vi "recipe_logic.vi"(5 "change_in_event":refnum<user-event>, 7 "transition_queue":refnum<queue>, 8 "error in (no error)":errorcluster, 11 "data_in":T1) -> (0 "error out":errorcluster, 1 "data out":variant, 2 "change":bool, 3 "data_out":T1)   [LabVIEW 2015, in "lv-recipe-machine.lvlib"]
uses:
  lv-recipe-machine.lvlib
  public/_controls/recipe_data.ctl
  public/_controls/mode.ctl
  public/_controls/manual_state.ctl
  public/_controls/automatic_state.ctl
  public/_controls/timer.ctl
  public/_controls/recipe_step.ctl
  public/_controls/change.ctl
  public/_controls/transition.ctl
  _controls/timers.ctl
  _controls/timer_command.ctl
  public/_controls/step.ctl
  public/_controls/error.ctl
  _controls/automatic_vi_variant_data.ctl
  <vilib>/ptbypt/NI_PtbyPt.lvlib
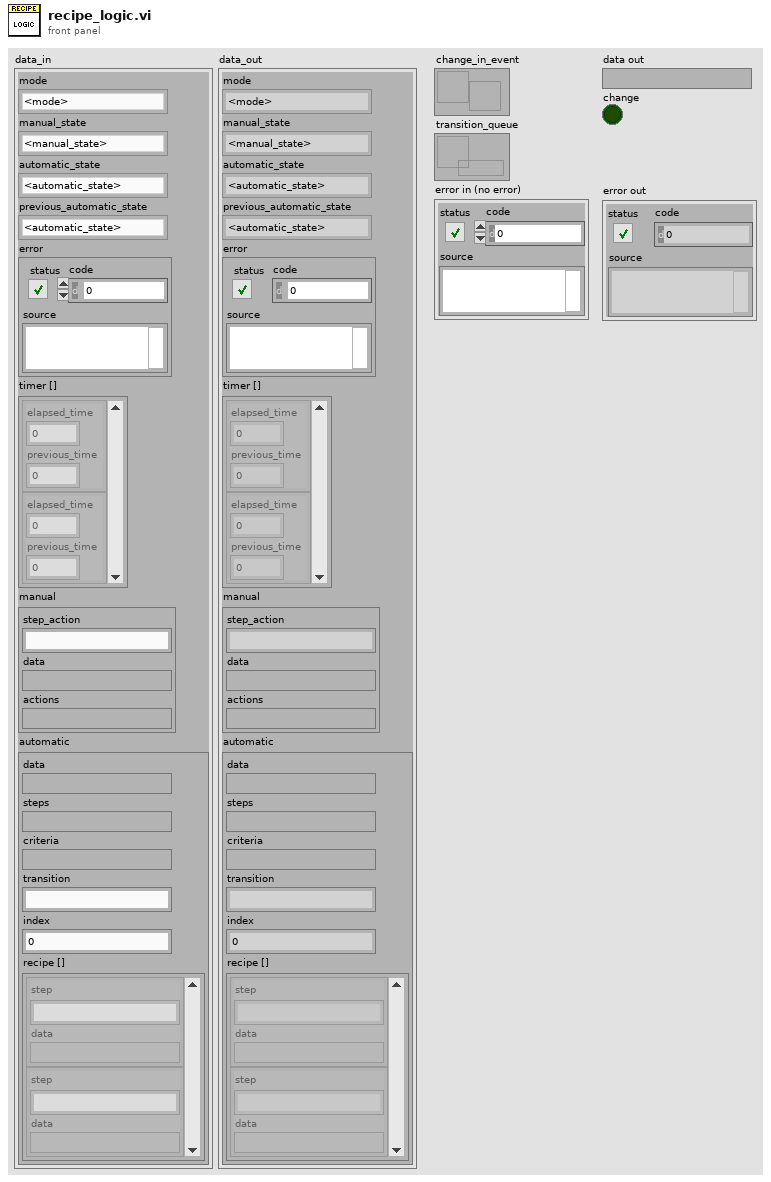
[diagram p1: front panel]
types:
  T1 = typedef "lv-recipe-machine.lvlib/recipe_data.ctl" = cluster{"mode":T2, "manual_state":T3, "automatic_state":T4, "previous_automatic_state":T4, "error":errorcluster, "timer []":T5[], "manual":cluster{"step_action":string, "data":variant, "actions":variant}, "automatic":cluster{"data":variant, "steps":variant, "criteria":variant, "transition":string, "index":i32, "recipe []":T6[]}}
  T2 = typedef "lv-recipe-machine.lvlib/mode.ctl" = enum16{"<mode>", "manual", "automatic", "<null>"}
  T3 = typedef "lv-recipe-machine.lvlib/manual_state.ctl" = enum16{"<manual_state>", "failed", "action", "running", "idle", "<null>"}
  T4 = typedef "lv-recipe-machine.lvlib/automatic_state.ctl" = enum16{"<automatic_state>", "failed", "idle", "running", "paused", "stopped", "<null>"}
  T5 = typedef "lv-recipe-machine.lvlib/timer.ctl" = cluster{"elapsed_time":dbl, "previous_time":dbl}
  T6 = typedef "lv-recipe-machine.lvlib/recipe_step.ctl" = cluster{"step":string, "data":variant}
  T7 = typedef "lv-recipe-machine.lvlib/timers.ctl" = enum16{"<timers>", "step", "recipe", "<null>"}
  T8 = typedef "lv-recipe-machine.lvlib/timer_command.ctl" = enum16{"<timer_command>", "start", "read", "pause", "resume", "stop", "<null>"}
  T9 = typedef "lv-recipe-machine.lvlib/automatic_vi_variant_data.ctl" = cluster{"current_state":T4, "previous_state":T4, "criteria":variant, "data":variant, "recipe_data":variant, "index":i32, "step":string, "steps":variant}
  T10 = typedef "lv-recipe-machine.lvlib/error.ctl" = enum16{"<error>", "bad_command", "command_queue_timeout", "stop_notifier_timeout", "die_command_timeout", "not_in_manual_mode", "not_in_automatic_mode", "not_in_automatic_idle", "not_in_automatic_running", "not_in_automatic_paused", "automatic_step_not_found", "manual_action_not_found", "automatic_not_transition_vi", "transition_step_not_found", "unsupported_vi_type", "<null>"}
  T11 = typedef "lv-recipe-machine.lvlib/step.ctl" = cluster{"name":string, "data":variant, "vi_reference":variant}
  T12 = cluster{"data":variant, "steps":variant, "criteria":variant, "transition":string, "index":i32, "recipe []":T6[]}
  T13 = cluster{"step_action":string, "data":variant, "actions":variant}
  T14 = typedef "lv-recipe-machine.lvlib/transition.ctl" = cluster{"next_index":i32, "data":variant, "recipe_data":variant, "error":errorcluster}
  T15 = cluster{"recipe_data out":variant, "error":errorcluster}
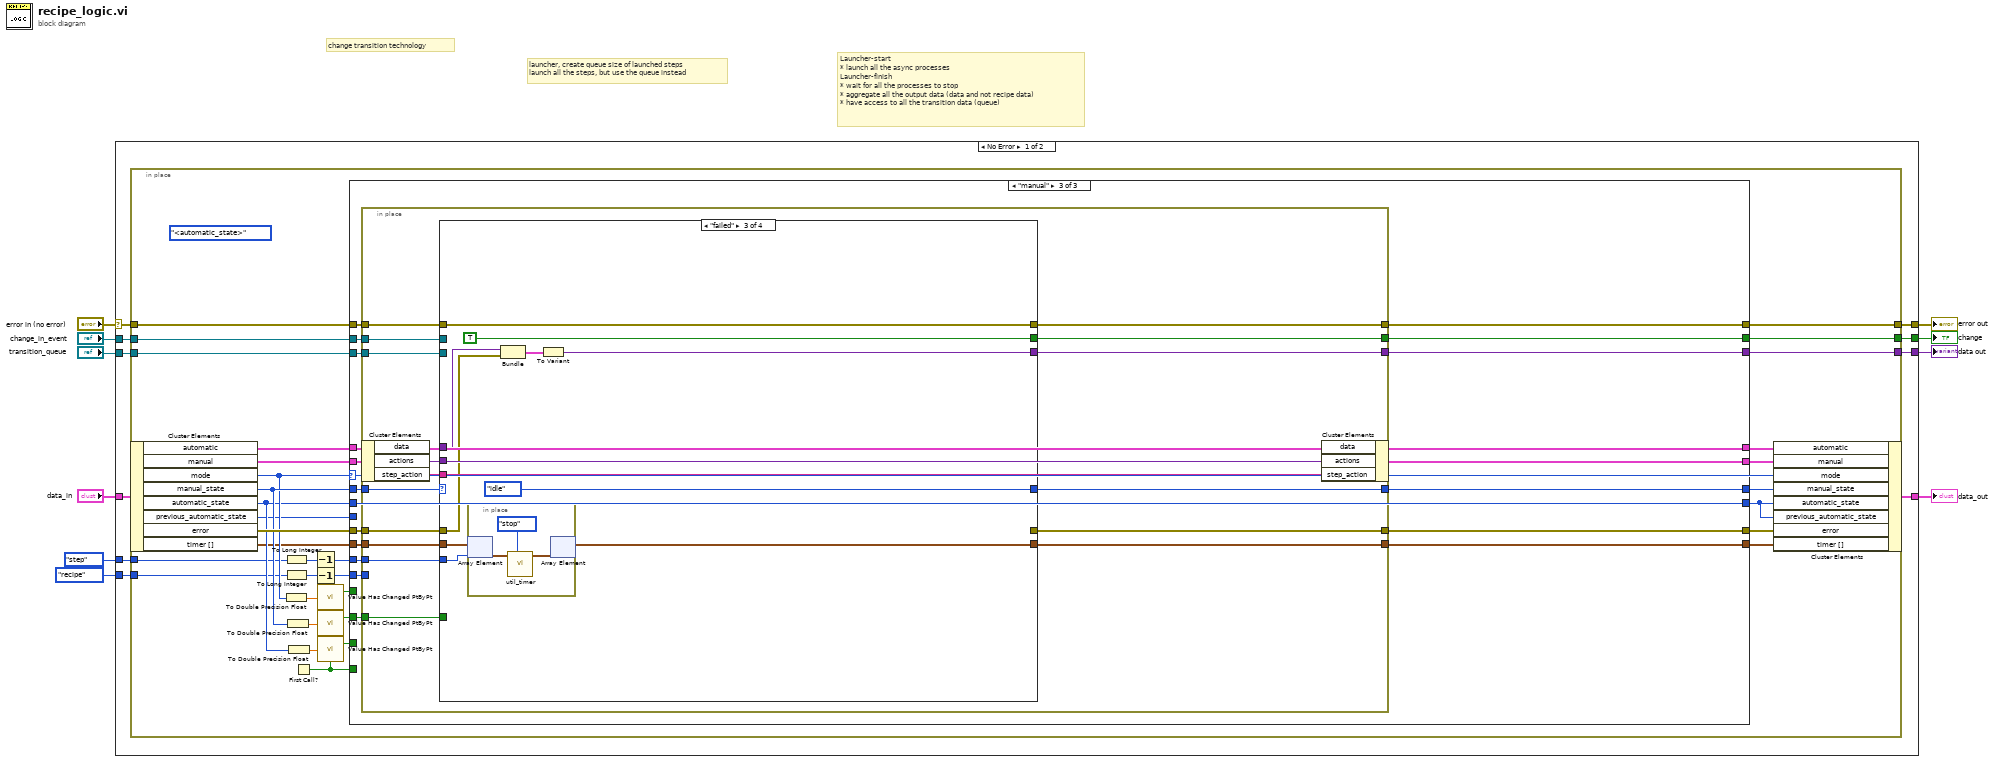
[diagram p0: block diagram]
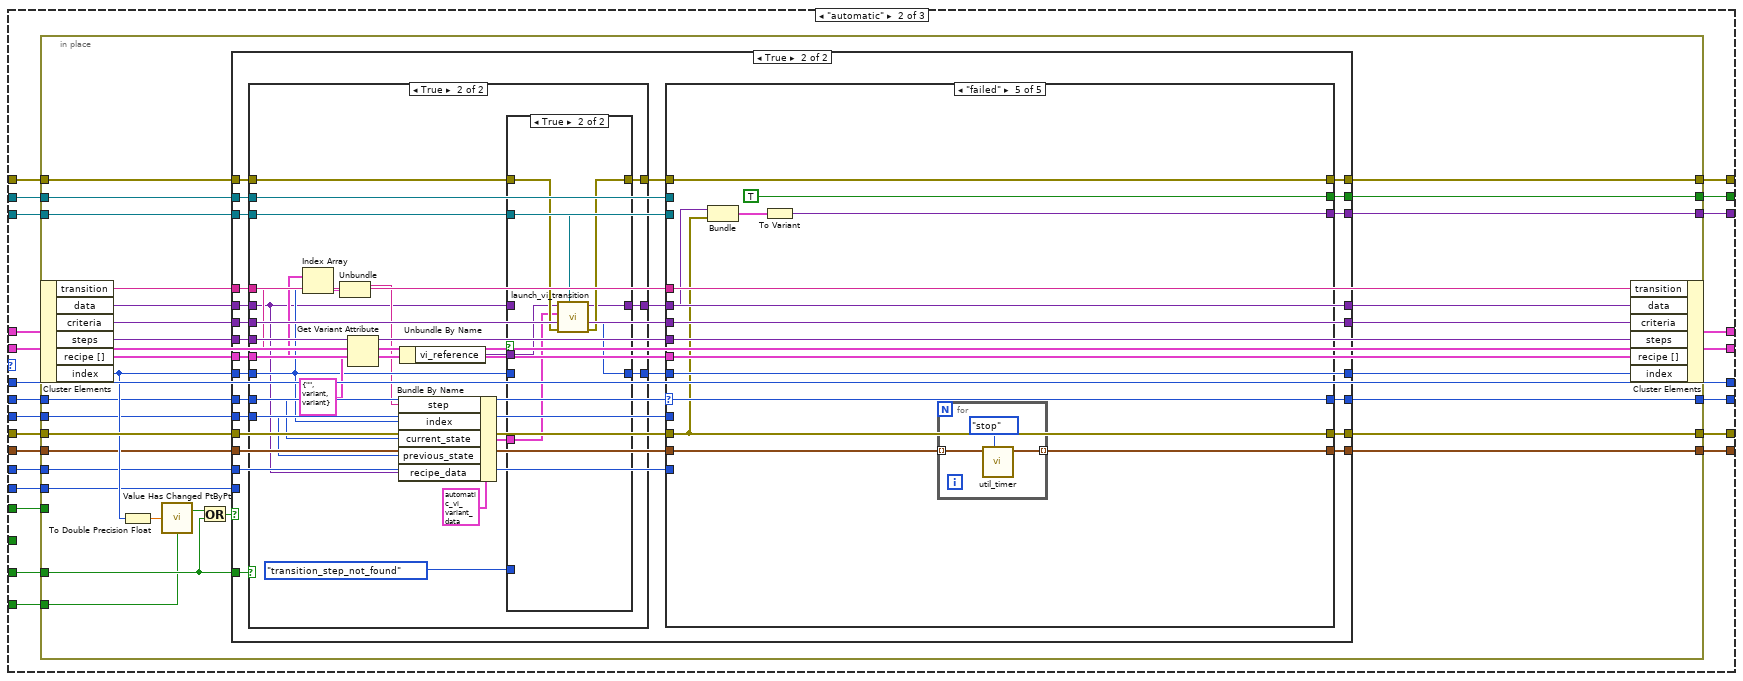
[diagram p3: hidden frame]
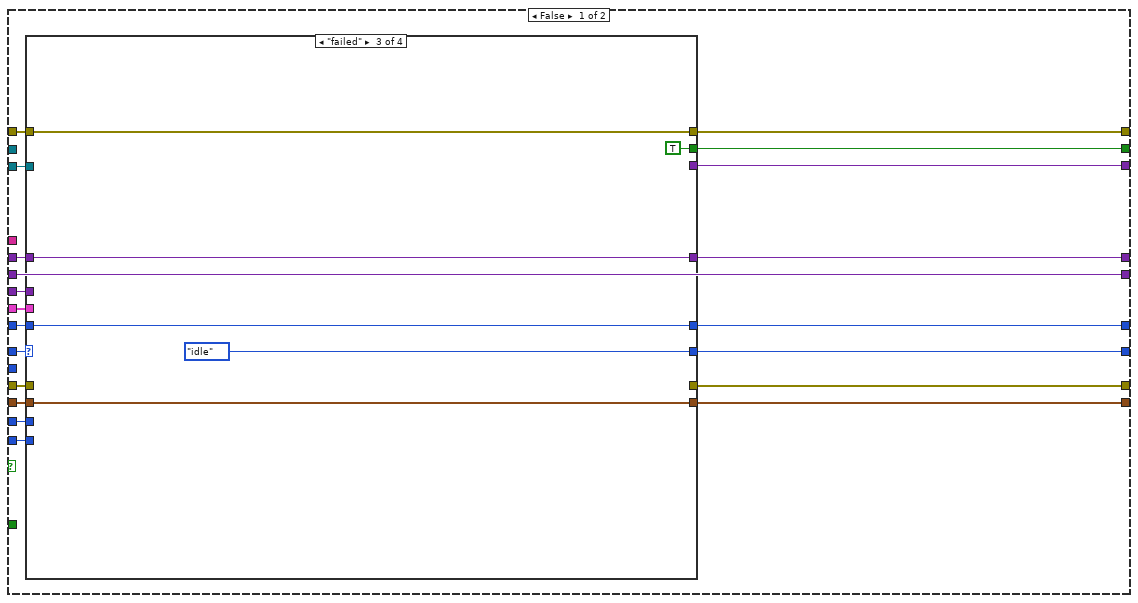
[diagram p4: hidden frame]
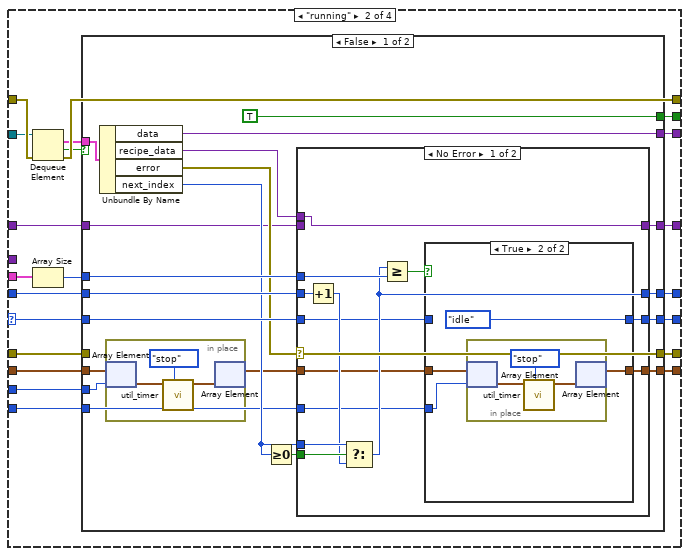
[diagram p6: hidden frame]
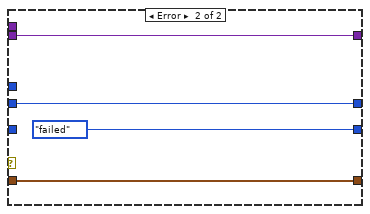
[diagram p8: hidden frame]
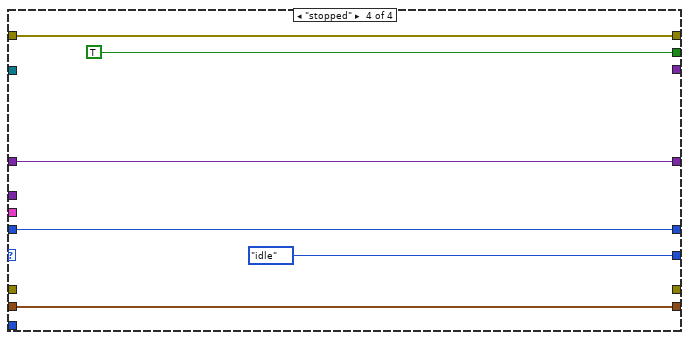
[diagram p10: hidden frame]
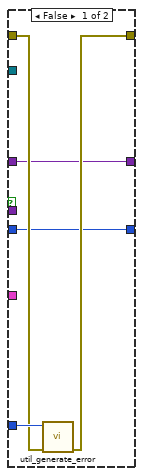
[diagram p12: hidden frame]
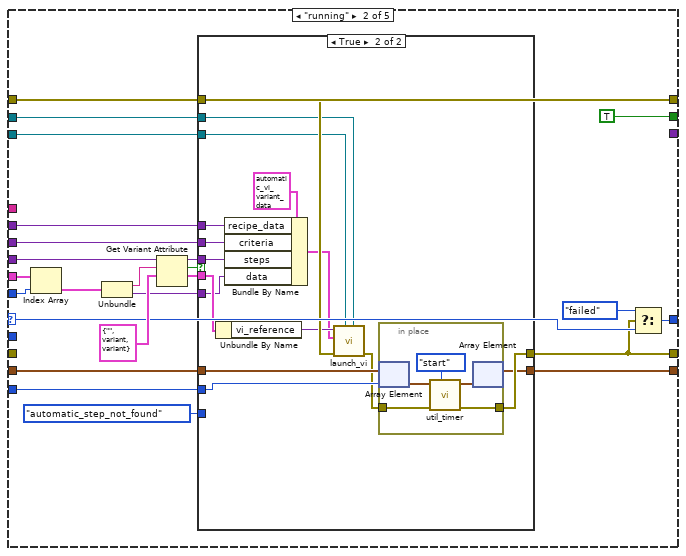
[diagram p14: hidden frame]
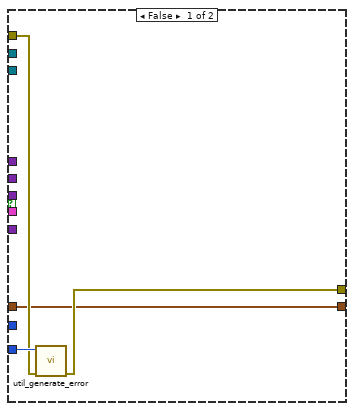
[diagram p15: hidden frame]
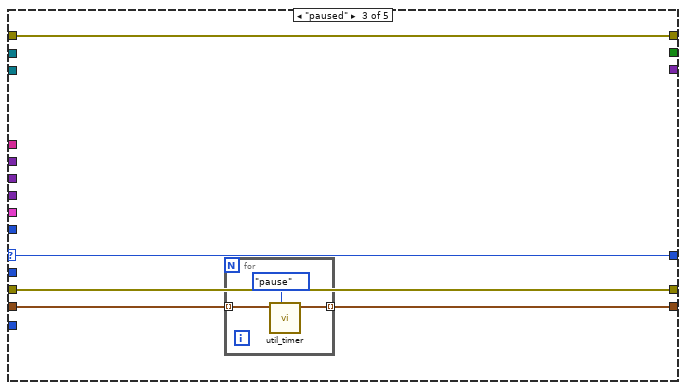
[diagram p16: hidden frame]
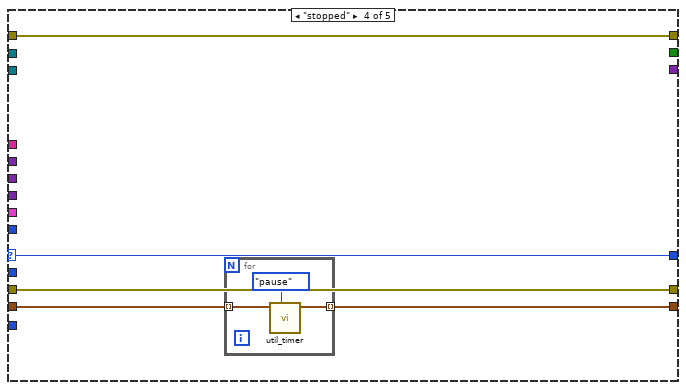
[diagram p17: hidden frame]
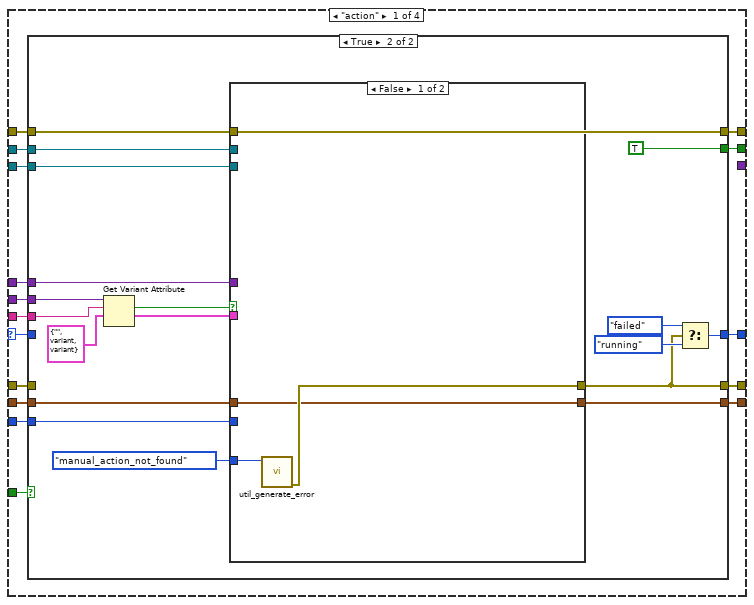
[diagram p18: hidden frame]
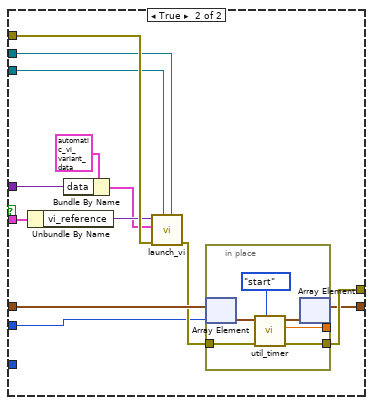
[diagram p20: hidden frame]
diagram:
  # "change transition technology"
  # "launcher, create queue size of launched steps\nlaunch all the steps, but use the queue instead"
  # "Launcher-start\n* launch all the async processes\nLauncher-finish\n* wait for all the processes to stop\n* aggregate all the output data (data and not recipe data)\n* have access to all the transition data (queue)"
  n1 = case shown="No Error" "error in (no error)" {
    selector: "error in (no error)" -> [w20 w512]
    tunnel: [w17 w512] -> w9
    tunnel: "data_in" -> [w19 w511]
    tunnel: [w18 w511] -> w7
    tunnel: [w16 _] -> w6
    tunnel: [w15 _] -> w5
    tunnel: "change_in_event" -> [w14 _]
    tunnel: "transition_queue" -> [w13 _]
    tunnel: timers."step" ("timers") -> [w12 _]
    tunnel: timers."recipe" ("timers") -> [w11 _]
    frame No Error {
      n2 = in-place {
        in-place-border: w20 -> [w46]
        in-place-border: [w43] -> w17
        in-place-border: [w40] -> w16
        in-place-border: [w39] -> w15
        in-place-border: w14 -> [w30]
        in-place-border: w13 -> [w29]
        in-place-border: w12 -> [w24]
        in-place-border: w11 -> [w23]
        (unwired) automatic_state."<automatic_state>" ("automatic_state")
        n3 = in-place-cluster #1(w19) -> ("automatic"=w35:T12, "manual"=w34:T13, "mode"=w42:T2, "manual_state"=w44:T3, "automatic_state"=w38:T4, "previous_automatic_state"=w37:T4, "error"=w53:errorcluster, "timer []"=w28:T5[])
        n4 = To Long Integer(number=w24) -> (32bit integer=w21:i32)
        n5 = To Long Integer(number=w23) -> (32bit integer=w22:i32)
        n6 = To Double Precision Float(number=w42) -> (double precision float=w52:dbl)
        n7 = To Double Precision Float(number=w44) -> (double precision float=w51:dbl)
        n8 = To Double Precision Float(number=w38) -> (double precision float=w50:dbl)
        n9 = First Call?() -> (First Call?: T/F=w45:bool)
        n10 = Decrement(x=w21) -> (x-1=w26:i32)
        n11 = Decrement(x=w22) -> (x-1=w25:i32)
        n12 = call <vilib>:"Value Has Changed PtByPt.vi"("input data point"=w52, "initialize"=w45) -> ("has changed"=w49:bool)  [unwired: 1 out]
        n13 = call <vilib>:"Value Has Changed PtByPt.vi"("input data point"=w51, "initialize"=w45) -> ("has changed"=w48:bool)  [unwired: 1 out]
        n14 = call <vilib>:"Value Has Changed PtByPt.vi"("input data point"=w50, "initialize"=w45) -> ("has changed"=w47:bool)  [unwired: 1 out]
        n15 = case shown="\"manual\"" w42 {
          tunnel: w44 -> [w59 w78 w383]
          tunnel: w38 -> [w58 w81 w378]
          tunnel: w49 -> [_ w61 _]
          tunnel: w48 -> [_ _ w382]
          tunnel: w47 -> [_ w77 _]
          tunnel: w45 -> [_ w74 _]
          tunnel: w46 -> [w60 w80 w381]
          tunnel: [w60 w79 w380] -> w43
          tunnel: [w59 w78 w379] -> w41
          tunnel: [w58 w71 w378] -> w31
          tunnel: [_ w73 w377] -> w40
          tunnel: [_ w72 w376] -> w39
          tunnel: w34 -> [w57 w82 w374]
          tunnel: w35 -> [w56 w76 w375]
          tunnel: [w56 w75 w375] -> w32
          tunnel: [w57 w82 w373] -> w33
          tunnel: w37 -> [_ w68 _]
          tunnel: w53 -> [w55 w70 w372]
          tunnel: [w55 w69 w371] -> w36
          tunnel: w30 -> [_ w67 w369]
          tunnel: w29 -> [_ w66 w370]
          tunnel: w28 -> [w54 w65 w366]
          tunnel: [w54 w62 w365] -> w27
          tunnel: w26 -> [_ w64 w368]
          tunnel: w25 -> [_ w63 w367]
          frame Default {
          }
          frame "automatic" {
            n16 = in-place {
              in-place-border: w81 -> [w90]
              in-place-border: w80 -> [w111]
              in-place-border: [w110] -> w79
              in-place-border: w77 -> [w92]
              in-place-border: w74 -> [w84]
              in-place-border: [w104] -> w73
              in-place-border: [w103] -> w72
              in-place-border: [w102] -> w71
              in-place-border: w70 -> [w99]
              in-place-border: [w98] -> w69
              in-place-border: w68 -> [w93]
              in-place-border: w67 -> [w89]
              in-place-border: w66 -> [w88]
              in-place-border: w65 -> [w87]
              in-place-border: w64 -> [w86]
              in-place-border: w63 -> [w85]
              in-place-border: [w83] -> w62
              in-place-border: w61 -> [_]
              n17 = in-place-cluster #2(w76) -> ("transition"=w94:string, "data"=w101:variant, "criteria"=w97:variant, "steps"=w107:variant, "recipe []"=w109:T6[], "index"=w96:i32)
              n18 = To Double Precision Float(number=w96) -> (double precision float=w108:dbl)
              n19 = call <vilib>:"Value Has Changed PtByPt.vi"("input data point"=w108, "initialize"=w84) -> ("has changed"=w106:bool)  [unwired: 1 out]
              n20 = Or(x=w106, y=w92) -> (x .or. y?=w105:bool)
              n21 = case shown="True" w105 {
                tunnel: w90 -> [w131 w238]
                tunnel: w111 -> [w130 w243]
                tunnel: [w129 w247] -> w110
                tunnel: w107 -> [w119 w236]
                tunnel: w96 -> [w128 w234]
                tunnel: w109 -> [w127 w230]
                tunnel: [w126 w246] -> w104
                tunnel: [w125 w224] -> w103
                tunnel: [w124 w245] -> w102
                tunnel: w101 -> [w123 w240]
                tunnel: [w122 w235] -> w100
                tunnel: w99 -> [w121 w233]
                tunnel: [w120 w244] -> w98
                tunnel: w97 -> [w118 w239]
                tunnel: [w118 w239] -> w95
                tunnel: w94 -> [_ w242]
                tunnel: w93 -> [_ w237]
                tunnel: w92 -> [_ w232]
                tunnel: [w117 w231] -> w91
                tunnel: w89 -> [_ w229]
                tunnel: w88 -> [w116 w228]
                tunnel: w87 -> [w115 w227]
                tunnel: w86 -> [w113 w226]
                tunnel: w85 -> [w112 _]
                tunnel: [w114 w225] -> w83
                frame False {
                  n22 = case shown="\"failed\"" w131 {
                    selector: w131 -> [w136 w153 _ _]
                    tunnel: w130 -> [w137 w158 w214 w223]
                    tunnel: [w137 w157 w214 w223] -> w129
                    tunnel: w119 -> [_ _ _ _]
                    tunnel: w128 -> [w133 w151 w215 w219]
                    tunnel: w127 -> [_ w150 _ _]
                    tunnel: [_ w155 TRUE TRUE] -> w126
                    tunnel: [_ w154 _ _] -> w125
                    tunnel: [w136 w152 automatic_state."idle" ("automatic_state") automatic_state."idle" ("automatic_state")] -> w124
                    tunnel: w123 -> [w135 w148 w216 w220]
                    tunnel: [w135 w147 w216 w220] -> w122
                    tunnel: w121 -> [w134 w156 _ _]
                    tunnel: [w134 w146 _ _] -> w120
                    tunnel: [w133 w145 w215 w219] -> w117
                    tunnel: w116 -> [_ w142 _ _]
                    tunnel: w115 -> [w132 w141 w213 w218]
                    tunnel: [w132 w139 w213 w218] -> w114
                    tunnel: w113 -> [_ w140 _ _]
                    tunnel: w112 -> [_ w138 _ _]
                    frame Default {
                    }
                    frame "running" {
                      n23 = Dequeue Element(queue=w142, error in (no error)=w158) -> (element=w144:T14, timed out?=w143:bool, error out=w157:errorcluster)  [unwired: 1 in, 1 out]
                      n24 = Array Size(array=w150) -> (size(s)=w149:i32)
                      n25 = case shown="False" w143 {
                        tunnel: [TRUE _] -> w155
                        tunnel: [w175 _] -> w154
                        tunnel: w153 -> [w172 w211]
                        tunnel: [w174 w211] -> w152
                        tunnel: w151 -> [w173 w208]
                        tunnel: w149 -> [w171 _]
                        tunnel: w144 -> [w176 _]
                        tunnel: w148 -> [w166 w210]
                        tunnel: [w165 w210] -> w147
                        tunnel: w156 -> [_ w209]
                        tunnel: [w170 w209] -> w146
                        tunnel: [w167 w208] -> w145
                        tunnel: w141 -> [w163 w207]
                        tunnel: w140 -> [w162 _]
                        tunnel: [w159 w207] -> w139
                        tunnel: w138 -> [w160 _]
                        frame False {
                          n26 = Unbundle By Name(w176) -> ("data"=w175:variant, "recipe_data"=w164:variant, "error"=w170:errorcluster, "next_index"=w169:i32)
                          n27 = in-place {
                            n28 = in-place-array #3(w163, w162) -> (w179:T5)
                            n29 = call "util_timer.vi"("timer_command"=timer_command."stop", "timer in"=w179) -> ("timer out"=w178:T5)  [unwired: 7 in, 2 out]
                            n30 = in-place-array #3(w178) -> (w161:T5[])  [unwired: 1 out]
                          }
                          n31 = Greater Or Equal To 0?(x=w169) -> (x >= 0?=w168:bool)
                          n32 = case shown="No Error" w170 {
                            tunnel: [w184 automatic_state."failed" ("t")] -> w174
                            tunnel: w173 -> [w192 w205]
                            tunnel: w172 -> [w185 _]
                            tunnel: w171 -> [w193 _]
                            tunnel: [w188 w205] -> w167
                            tunnel: w169 -> [w190 _]
                            tunnel: w168 -> [w191 _]
                            tunnel: w166 -> [_ w204]
                            tunnel: [w187 w204] -> w165
                            tunnel: w164 -> [w187 _]
                            tunnel: w161 -> [w183 w203]
                            tunnel: w160 -> [w182 _]
                            tunnel: [w181 w203] -> w159
                            frame No Error {
                              n33 = Increment(x=w192) -> (x+1=w189:i32)
                              n34 = Select(t=w190, s=w191, f=w189) -> (s? t:f=w188:i32)
                              n35 = Greater Or Equal?(x=w188, y=w193) -> (x >= y?=w186:bool)
                              n36 = case shown="True" w186 {
                                tunnel: w185 -> [w195 _]
                                tunnel: [w195 automatic_state."idle" ("t")] -> w184
                                tunnel: w183 -> [w194 w198]
                                tunnel: w182 -> [_ w197]
                                tunnel: [w194 w196] -> w181
                                frame False {
                                }
                                frame True {
                                n37 = in-place {
                                n38 = in-place-array #4(w198, w197) -> (w201:T5)
                                n39 = call "util_timer.vi"("timer_command"=timer_command."stop", "timer in"=w201) -> ("timer out"=w200:T5)  [unwired: 7 in, 2 out]
                                n40 = in-place-array #4(w200) -> (w196:T5[])  [unwired: 1 out]
                                }
                                }
                              }
                            }
                            frame Error {
                            }
                          }
                        }
                        frame True {
                        }
                      }
                    }
                    frame "failed" {
                    }
                    frame "stopped" {
                    }
                  }
                }
                frame True {
                  n41 = case shown="True" w232 {
                    tunnel: w243 -> [w250 w271]
                    tunnel: [w250 w270] -> w241
                    tunnel: w240 -> [w248 w252]
                    tunnel: w239 -> [_ _]
                    tunnel: w238 -> [_ w255]
                    tunnel: w237 -> [_ w254]
                    tunnel: w236 -> [_ w269]
                    tunnel: [w248 w264] -> w235
                    tunnel: w234 -> [w249 w257]
                    tunnel: [w249 w263] -> w231
                    tunnel: w242 -> [_ w268]
                    tunnel: w230 -> [_ w258]
                    tunnel: w229 -> [_ _]
                    tunnel: w228 -> [_ w251]
                    frame False {
                    }
                    frame True {
                      n42 = Index Array(array=w258, index=w257) -> (element=w256:T6)
                      n43 = Unbundle(w256) -> ("step"=w253:string)  [unwired: 1 out]
                      n44 = Get Variant Attribute(Variant=w269, name=w268, default value (empty Variant)=T11 {"name"="", "data"=variant, "vi_reference"=variant(refnum<vi> refnum)} ("step")) -> (found=w261:bool, value=w266:T11)  [unwired: 1 in, 2 out]
                      n45 = Bundle By Name(cluster=T9 {"current_state"=enum."<automatic_state>", "previous_state"=enum."<automatic_state>", "criteria"=variant, "data"=variant, "recipe_data"=variant, "index"=0, "step"="", "steps"=variant} ("data"), "step"=w253, "index"=w257, "current_state"=w255, "previous_state"=w254, "recipe_data"=w252) -> (w259:T9)
                      n46 = Unbundle By Name(w266) -> ("vi_reference"=w265:variant)
                      n47 = case shown="True" w261 {
                        tunnel: w271 -> [w275 w283]
                        tunnel: [w274 w282] -> w270
                        tunnel: w265 -> [_ w281]
                        tunnel: w252 -> [w273 _]
                        tunnel: [w273 w278] -> w264
                        tunnel: w257 -> [w272 _]
                        tunnel: [w272 w280] -> w263
                        tunnel: error."transition_step_not_found" ("error") -> [w276 _]
                        tunnel: w259 -> [_ w279]
                        tunnel: w251 -> [_ w277]
                        frame False {
                          n48 = call "util_generate_error.vi"("error in (no error)"=w275, "error"=w276) -> ("error out"=w274:errorcluster)  [unwired: 9 in]
                        }
                        frame True {
                          n49 = call "launch_vi_transition.vi"("transition_queue"=w277, "error in (no error)"=w283, "data"=w279, "vi_reference"=w281) -> ("error out"=w282:errorcluster, "index out"=w280:i32, "recipe_data out"=w278:variant)  [unwired: 5 in]
                        }
                      }
                    }
                  }
                  n50 = case shown="\"failed\"" w238 {
                    selector: w238 -> [w286 w305 w339 w347 w358]
                    tunnel: w241 -> [w287 w297 w337 w345 w353]
                    tunnel: [w287 w297 w337 w345 w353] -> w247
                    tunnel: [w286 w308 w339 w347 w358] -> w245
                    tunnel: [_ TRUE _ _ TRUE] -> w246
                    tunnel: w236 -> [_ w306 _ _ _]
                    tunnel: w231 -> [_ w302 _ _ _]
                    tunnel: w230 -> [_ w303 _ _ _]
                    tunnel: w235 -> [_ w294 _ _ w355]
                    tunnel: [w285 w296 w338 w346 w356] -> w244
                    tunnel: w239 -> [_ w295 _ _ _]
                    tunnel: w242 -> [_ _ _ _ _]
                    tunnel: w237 -> [_ _ _ _ _]
                    tunnel: w233 -> [w285 _ w338 w346 w356]
                    tunnel: w229 -> [_ w292 _ _ _]
                    tunnel: w228 -> [_ w291 _ _ _]
                    tunnel: w227 -> [w284 w290 w341 w349 w360]
                    tunnel: w226 -> [_ w289 _ _ _]
                    tunnel: [w284 w288 w340 w348 w359] -> w225
                    tunnel: [_ _ _ _ w354] -> w224
                    frame Default {
                    }
                    frame "running" {
                      n51 = Index Array(array=w303, index=w302) -> (element=w301:T6)
                      n52 = Unbundle(w301) -> ("step"=w300:string, "data"=w299:variant)
                      n53 = Get Variant Attribute(Variant=w306, name=w300, default value (empty Variant)=T11 {"name"="", "data"=variant, "vi_reference"=variant(refnum<vi> refnum)} ("step")) -> (duplicate Variant=w293:variant, found=w309:bool, value=w310:T11)  [unwired: 1 in, 1 out]
                      n54 = case shown="True" w309 {
                        tunnel: w310 -> [_ w330]
                        tunnel: w299 -> [_ w324]
                        tunnel: error."automatic_step_not_found" ("error") -> [w315 _]
                        tunnel: w297 -> [w314 w331]
                        tunnel: [w313 w317] -> w296
                        tunnel: w295 -> [_ w326]
                        tunnel: w294 -> [_ w325]
                        tunnel: w293 -> [_ w323]
                        tunnel: w292 -> [_ w322]
                        tunnel: w291 -> [_ w321]
                        tunnel: w290 -> [w312 w320]
                        tunnel: w289 -> [_ w319]
                        tunnel: [w312 w316] -> w288
                        frame False {
                          n55 = call "util_generate_error.vi"("error in (no error)"=w314, "error"=w315) -> ("error out"=w313:errorcluster)  [unwired: 9 in]
                        }
                        frame True {
                          n56 = Unbundle By Name(w330) -> ("vi_reference"=w329:variant)
                          n57 = Bundle By Name(cluster=T9 {"current_state"=enum."<automatic_state>", "previous_state"=enum."<automatic_state>", "criteria"=variant, "data"=variant, "recipe_data"=variant, "index"=0, "step"="", "steps"=variant} ("data"), "recipe_data"=w325, "criteria"=w326, "steps"=w323, "data"=w324) -> (w328:T9)
                          n58 = call "launch_vi.vi"("change_in_event"=w322, "transition_queue"=w321, "error in (no error)"=w331, "data"=w328, "vi_reference"=w329) -> ("error out"=w318:errorcluster)  [unwired: 6 in]
                          n59 = in-place {
                            in-place-border: w318 -> [w333]
                            in-place-border: [w332] -> w317
                            n60 = in-place-array #5(w320, w319) -> (w335:T5)
                            n61 = call "util_timer.vi"("timer_command"=timer_command."start", "error in (no error)"=w333, "timer in"=w335) -> ("error out"=w332:errorcluster, "timer out"=w334:T5)  [unwired: 6 in, 1 out]
                            n62 = in-place-array #5(w334) -> (w316:T5[])  [unwired: 1 out]
                          }
                        }
                      }
                      n63 = Select(t=automatic_state."failed", s=w296, f=w305) -> (s? t:f=w308:T4)
                    }
                    frame "paused" {
                      n64 = for {
                        tunnel: w341 -> [w344] mode=indexing
                        tunnel: [w343] -> w340 mode=indexing
                        n65 = call "util_timer.vi"("timer_command"=timer_command."pause", "timer in"=w344) -> ("timer out"=w343:T5)  [unwired: 7 in, 2 out]
                      }
                    }
                    frame "stopped" {
                      n66 = for {
                        tunnel: w349 -> [w352] mode=indexing
                        tunnel: [w351] -> w348 mode=indexing
                        n67 = call "util_timer.vi"("timer_command"=timer_command."pause", "timer in"=w352) -> ("timer out"=w351:T5)  [unwired: 7 in, 2 out]
                      }
                    }
                    frame "failed" {
                      n68 = Bundle("recipe_data out"=w355, "error"=w356) -> (w361:T15)  [unwired: 1 in]
                      n69 = To Variant(anything=w361) -> (Variant=w354:variant)
                      n70 = for {
                        tunnel: w360 -> [w364] mode=indexing
                        tunnel: [w363] -> w359 mode=indexing
                        n71 = call "util_timer.vi"("timer_command"=timer_command."stop", "timer in"=w364) -> ("timer out"=w363:T5)  [unwired: 7 in, 2 out]
                      }
                    }
                  }
                }
              }
              n72 = in-place-cluster #2("transition"=w94, "data"=w100, "criteria"=w95, "steps"=w107, "recipe []"=w109, "index"=w91) -> (w75:T12)
            }
          }
          frame "manual" {
            n73 = in-place {
              in-place-border: w383 -> [w400]
              in-place-border: w382 -> [w399]
              in-place-border: w381 -> [w398]
              in-place-border: [w397] -> w380
              in-place-border: [w396] -> w379
              in-place-border: [w395] -> w377
              in-place-border: [w394] -> w376
              in-place-border: w372 -> [w390]
              in-place-border: [w389] -> w371
              in-place-border: w370 -> [w388]
              in-place-border: w369 -> [w387]
              in-place-border: w368 -> [w386]
              in-place-border: w367 -> [_]
              in-place-border: w366 -> [w385]
              in-place-border: [w384] -> w365
              n74 = in-place-cluster #6(w374) -> ("data"=w393:variant, "actions"=w392:variant, "step_action"=w391:string)
              n75 = case shown="\"failed\"" w400 {
                selector: w400 -> [w411 w472 _ w509]
                tunnel: w391 -> [w408 _ _ _]
                tunnel: w398 -> [w416 w465 w503 w510]
                tunnel: [w415 w474 w503 w510] -> w397
                tunnel: [w414 w473 manual_state."idle" ("manual_state") w509] -> w396
                tunnel: [w413 w471 TRUE _] -> w395
                tunnel: [_ w470 w501 _] -> w394
                tunnel: w399 -> [w412 _ _ _]
                tunnel: w392 -> [w410 _ _ _]
                tunnel: w393 -> [w409 _ w497 _]
                tunnel: [w407 w469 _ _] -> w389
                tunnel: w390 -> [w406 w468 w496 _]
                tunnel: w388 -> [w405 w464 _ _]
                tunnel: w387 -> [w404 _ _ _]
                tunnel: w386 -> [w403 w462 w499 _]
                tunnel: w385 -> [w402 w463 w500 w508]
                tunnel: [w401 w461 w498 w508] -> w384
                frame "action" {
                  n76 = case shown="True" w412 {
                    tunnel: w416 -> [w420 w422]
                    tunnel: [w420 w422] -> w415
                    tunnel: [w419 w433] -> w414
                    tunnel: [_ TRUE] -> w413
                    tunnel: w408 -> [_ w431]
                    tunnel: w411 -> [w419 _]
                    tunnel: w410 -> [_ w430]
                    tunnel: w409 -> [_ w429]
                    tunnel: [w418 w427] -> w407
                    tunnel: w406 -> [w418 _]
                    tunnel: w405 -> [_ w426]
                    tunnel: w404 -> [_ w425]
                    tunnel: w403 -> [_ w424]
                    tunnel: w402 -> [w417 w423]
                    tunnel: [w417 w421] -> w401
                    frame False {
                    }
                    frame True {
                      n77 = Get Variant Attribute(Variant=w430, name=w431, default value (empty Variant)=T11 {"name"="", "data"=variant, "vi_reference"=variant(refnum<vi> refnum)} ("step")) -> (found=w436:bool, value=w437:T11)  [unwired: 1 in, 2 out]
                      n78 = case shown="False" w436 {
                        tunnel: w437 -> [_ w453]
                        tunnel: [w440 w444] -> w427
                        tunnel: w429 -> [_ w449]
                        tunnel: error."manual_action_not_found" ("error") -> [w441 _]
                        tunnel: w426 -> [_ w448]
                        tunnel: w425 -> [_ w447]
                        tunnel: w424 -> [_ w442]
                        tunnel: w423 -> [w439 w446]
                        tunnel: w422 -> [_ w454]
                        tunnel: [w439 w443] -> w421
                        frame False {
                          n79 = call "util_generate_error.vi"("error"=w441) -> ("error out"=w440:errorcluster)  [unwired: 10 in]
                        }
                        frame True {
                          n80 = Unbundle By Name(w453) -> ("vi_reference"=w452:variant)
                          n81 = Bundle By Name(cluster=T9 {"current_state"=enum."<automatic_state>", "previous_state"=enum."<automatic_state>", "criteria"=variant, "data"=variant, "recipe_data"=variant, "index"=0, "step"="", "steps"=variant} ("data"), "data"=w449) -> (w450:T9)
                          n82 = call "launch_vi.vi"("change_in_event"=w447, "transition_queue"=w448, "error in (no error)"=w454, "data"=w450, "vi_reference"=w452) -> ("error out"=w445:errorcluster)  [unwired: 6 in]
                          n83 = in-place {
                            in-place-border: w445 -> [w458]
                            in-place-border: [w457] -> w444
                            in-place-border: [w455] -> _
                            n84 = in-place-array #7(w446, w442) -> (w460:T5)
                            n85 = call "util_timer.vi"("timer_command"=timer_command."start", "error in (no error)"=w458, "timer in"=w460) -> ("error out"=w457:errorcluster, "elapsed_time"=w455:dbl, "timer out"=w459:T5)  [unwired: 6 in]
                            n86 = in-place-array #7(w459) -> (w443:T5[])  [unwired: 1 out]
                          }
                        }
                      }
                      n87 = Select(t=manual_state."failed" ("manual_state"), s=w427, f=manual_state."running" ("manual_state")) -> (s? t:f=w433:T3)
                    }
                  }
                }
                frame "running" {
                  n88 = Dequeue Element(queue=w464, error in (no error)=w465) -> (element=w467:T14, timed out?=w466:bool, error out=w474:errorcluster)  [unwired: 1 in, 1 out]
                  n89 = case shown="False" w466 {
                    tunnel: w467 -> [w485 _]
                    tunnel: [w484 w494] -> w473
                    tunnel: w472 -> [_ w494]
                    tunnel: [TRUE _] -> w471
                    tunnel: [w480 _] -> w470
                    tunnel: [w476 w493] -> w469
                    tunnel: w468 -> [_ w493]
                    tunnel: w463 -> [w479 w492]
                    tunnel: w462 -> [w478 _]
                    tunnel: [w475 w492] -> w461
                    frame False {
                      n90 = Unbundle By Name(w485) -> ("data"=w480:variant, "error"=w477:errorcluster)
                      n91 = in-place {
                        in-place-border: w477 -> [w488]
                        in-place-border: [w487] -> w476
                        in-place-border: [w486] -> _
                        n92 = in-place-array #8(w479, w478) -> (w491:T5)
                        n93 = call "util_timer.vi"("timer_command"=timer_command."stop", "error in (no error)"=w488, "timer in"=w491) -> ("error out"=w487:errorcluster, "elapsed_time"=w486:dbl, "timer out"=w490:T5)  [unwired: 6 in]
                        n94 = in-place-array #8(w490) -> (w475:T5[])  [unwired: 1 out]
                      }
                      n95 = Select(t=manual_state."failed" ("manual_state"), s=w476, f=manual_state."idle" ("manual_state")) -> (s? t:f=w484:T3)
                    }
                    frame True {
                    }
                  }
                }
                frame "failed" {
                  n96 = in-place {
                    n97 = in-place-array #9(w500, w499) -> (w506:T5)
                    n98 = call "util_timer.vi"("timer_command"=timer_command."stop", "timer in"=w506) -> ("timer out"=w505:T5)  [unwired: 7 in, 2 out]
                    n99 = in-place-array #9(w505) -> (w498:T5[])  [unwired: 1 out]
                  }
                  n100 = Bundle("data"=w497, "error"=w496) -> (w495:cluster{"data":variant, "error":errorcluster})  [unwired: 1 in]
                  n101 = To Variant(anything=w495) -> (Variant=w501:variant)
                }
                frame Default {
                }
              }
              n102 = in-place-cluster #6("data"=w393, "actions"=w392, "step_action"=w391) -> (w373:T13)
            }
          }
        }
        n103 = in-place-cluster #1("automatic"=w32, "manual"=w33, "mode"=w42, "manual_state"=w41, "automatic_state"=w31, "previous_automatic_state"=w31, "error"=w36, "timer []"=w27) -> (w18:T1)
      }
    }
    frame Error {
    }
  }
  "error out" <- w9
  "data_out" <- w7
  "change" <- w6
  "data out" <- w5
